vi "motor_temperatures.vi"() -> ()   [LabVIEW 2019]
panel:
  in  "stop":bool
  out "cluster":T1
  out "cancelled":bool
  in  "error in":errorcluster
  out "error out":errorcluster
  out "text":string[](array[string])
  out "T12":dbl
  out "T11":dbl
  out "T10":dbl
  out "T09":dbl
  out "T08":dbl
  out "T07":dbl
  out "T06":dbl
  out "T05":dbl
  out "T04":dbl
  out "T03":dbl
  out "T02":dbl
  out "T01":i32
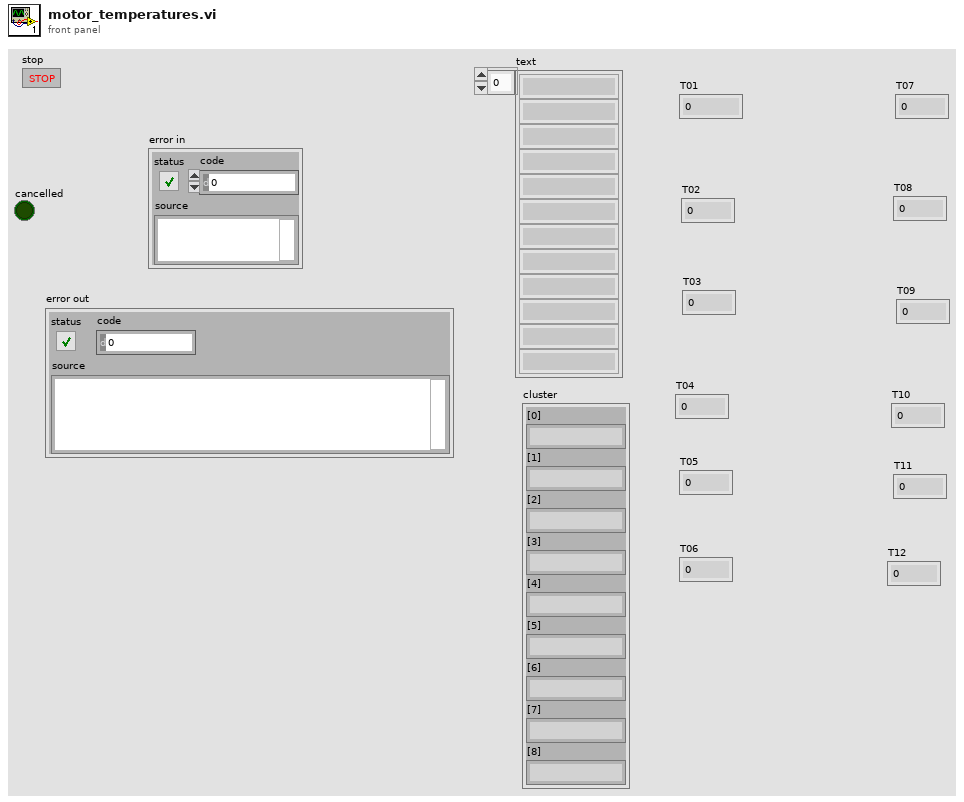
[diagram p1: front panel]
types:
  T1 = cluster{"[0]":string, "[1]":string, "[2]":string, "[3]":string, "[4]":string, "[5]":string, "[6]":string, "[7]":string, "[8]":string}
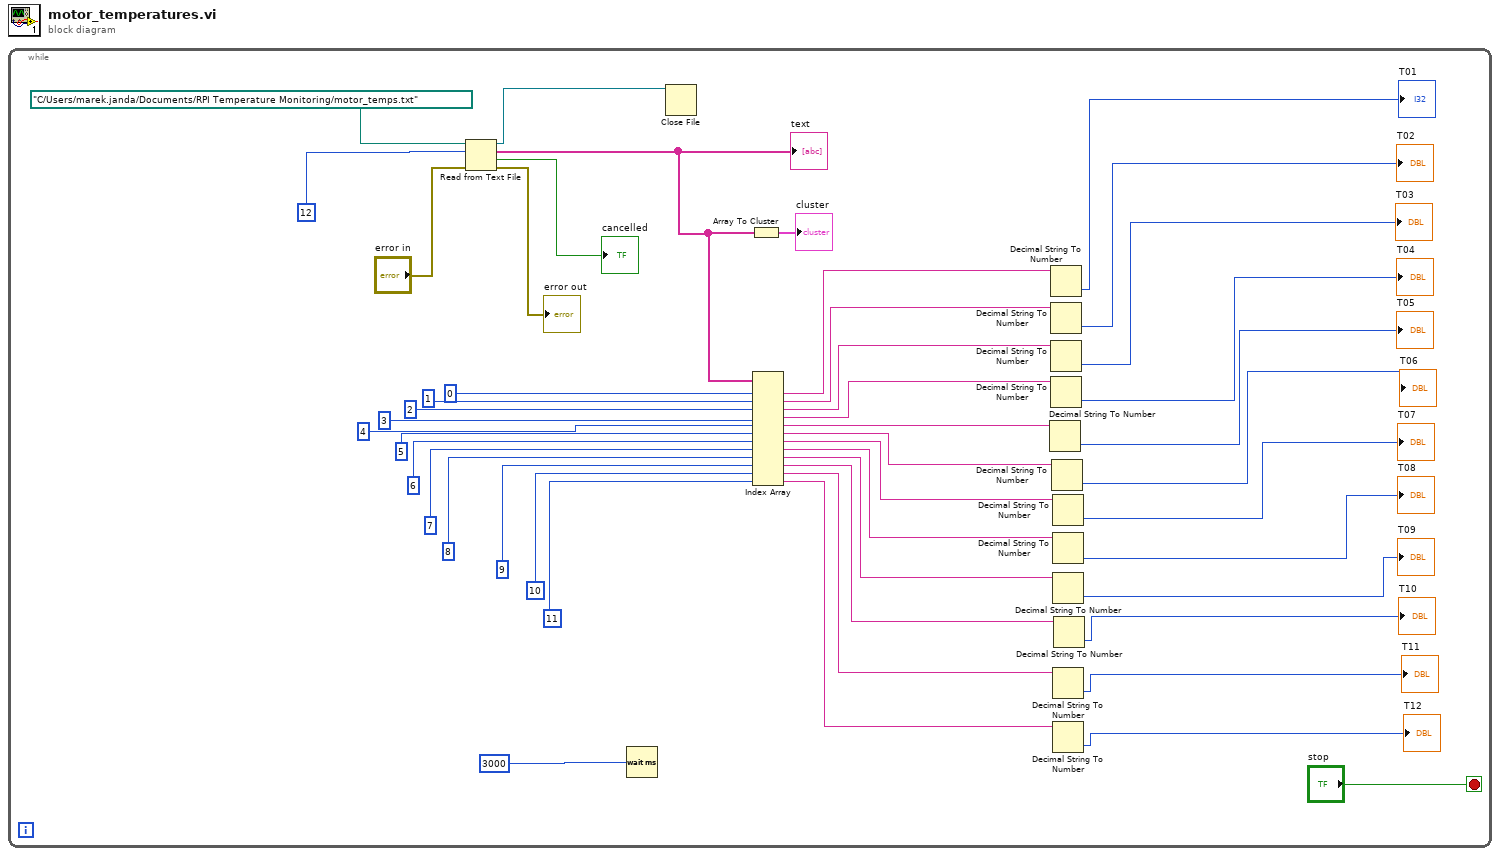
[diagram p0: block diagram]
diagram:
  n1 = while {
    stop <- "stop" stop-if-true
    n2 = Read from Text File(file (use dialog)=path "C:/Users/marek.janda/Documents/RPI Temperature Monitoring/motor_temps.txt", count=12, error in="error in") -> (refnum out=w14:refnum<file>, text=w41:string[], cancelled=→"cancelled":bool, error out=→"error out":errorcluster)  [unwired: 1 in]
    "text" <- w41
    n3 = Wait (ms)(milliseconds to wait=u32 3000) -> ()  [unwired: 1 out]
    n4 = Close File(refnum=w14) -> ()  [unwired: 1 in, 2 out]
    n5 = Array To Cluster(array=w41) -> (cluster=→"cluster":T1)
    n6 = Index Array(array=w41, index #1=0 ("index"), index #2=1 ("index"), index #3=2 ("index"), index #4=3 ("index"), index #5=4 ("index"), index #6=5 ("index"), index #7=6 ("index"), index #8=7 ("index"), index #9=8 ("index"), index #10=9 ("index"), index #11=10 ("index"), index #12=11 ("index")) -> (element #1=w28:string, element #2=w27:string, element #3=w26:string, element #4=w25:string, element #5=w24:string, element #6=w23:string, element #7=w22:string, element #8=w21:string, element #9=w20:string, element #10=w19:string, element #11=w18:string, element #12=w17:string)
    n7 = Decimal String To Number(string=w24) -> (number=→"T05":i32)  [unwired: 2 in, 1 out]
    n8 = Decimal String To Number(string=w28) -> (number=→"T01":i32)  [unwired: 2 in, 1 out]
    n9 = Decimal String To Number(string=w27) -> (number=→"T02":i32)  [unwired: 2 in, 1 out]
    n10 = Decimal String To Number(string=w26) -> (number=→"T03":i32)  [unwired: 2 in, 1 out]
    n11 = Decimal String To Number(string=w25) -> (number=→"T04":i32)  [unwired: 2 in, 1 out]
    n12 = Decimal String To Number(string=w23) -> (number=→"T06":i32)  [unwired: 2 in, 1 out]
    n13 = Decimal String To Number(string=w22) -> (number=→"T07":i32)  [unwired: 2 in, 1 out]
    n14 = Decimal String To Number(string=w21) -> (number=→"T08":i32)  [unwired: 2 in, 1 out]
    n15 = Decimal String To Number(string=w20) -> (number=→"T09":i32)  [unwired: 2 in, 1 out]
    n16 = Decimal String To Number(string=w18) -> (number=→"T11":i32)  [unwired: 2 in, 1 out]
    n17 = Decimal String To Number(string=w17) -> (number=→"T12":i32)  [unwired: 2 in, 1 out]
    n18 = Decimal String To Number(string=w19) -> (number=→"T10":i32)  [unwired: 2 in, 1 out]
  }
